vi "JKISM++ Start Async Call.vi"   [LabVIEW 2014, in "JKI State Machine++.lvlib"]
doc: "异步调用模板代码的VI片段\n\n<b>输入控件:</b>\n - 无\n\n<b>输出控件:</b>\n - 无"
uses:
  JKI State Machine++.lvlib
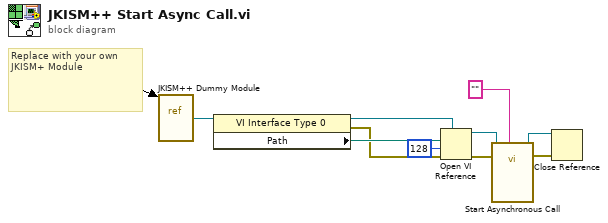
[diagram p0: block diagram]
diagram:
  # "Replace with your own JKISM+ Module"
  n1 = vi-ref "JKISM++ Dummy Module.vi"() -> (w9:refnum<vi>)
  n2 = property class="VI Interface Type 0"(reference=w9) -> (reference out=w5:refnum<vi>, error out=w7:errorcluster, "Path"=w8:path)  [unwired: 1 in]
  n3 = Open VI Reference(type specifier VI Refnum (for type only)=w5, vi path=w8, options=128, error in (no error)=w7) -> (vi reference=w6:refnum<vi>, error out=w10:errorcluster)  [unwired: 2 in]
  n4 = call-by-ref "Start Asynchronous Call"(reference=w6, error in=w10, "Name(\"\" to use uuid)"="" ("Name(\"\" to use uuid)")) -> (reference out=w2:refnum<vi>, error out=w3:errorcluster)  [unwired: 11 in]
  n5 = Close Reference(reference=w2, error in (no error)=w3) -> ()  [unwired: 1 out]
